vi "AnalysisCompleted.vi"(0 "SystemEvents in":refnum<class "SystemEvents.lvclass">, 1 "event data":variant, 5 "error in (no error)":errorcluster) -> (14 "SystemEvents out":refnum<class "SystemEvents.lvclass">, 19 "error out":errorcluster)   [LabVIEW 2017, in "SystemEvents.lvclass"]
doc: "Fires the Analysis completed event."
uses:
  SystemEvents.lvclass
  SystemEvents.lvclass/SystemEvents.ctl
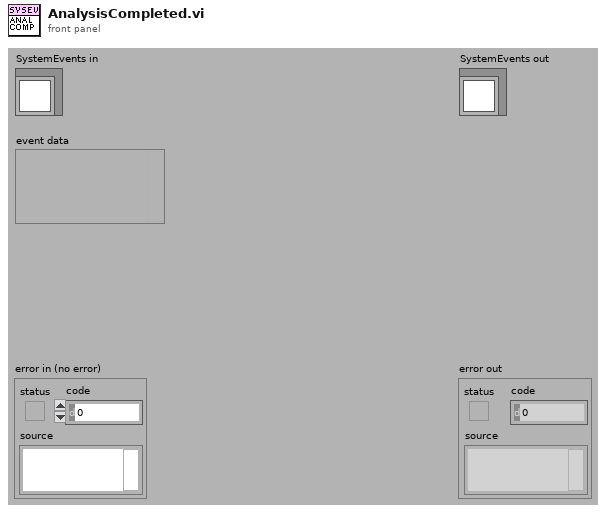
[diagram p1: front panel]
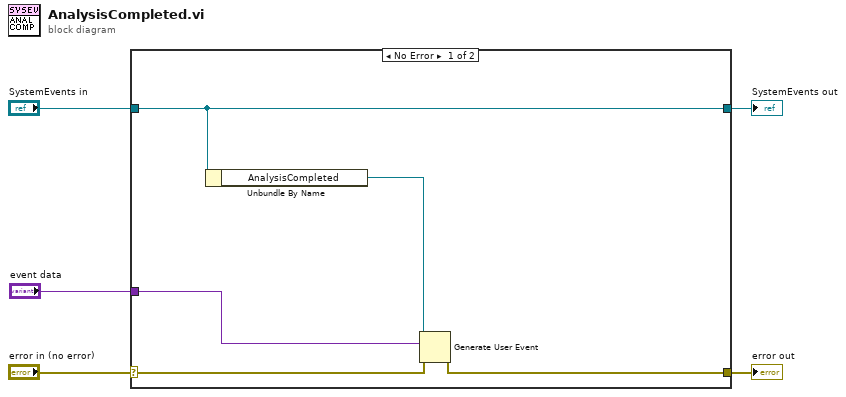
[diagram p0: block diagram]
diagram:
  n1 = case shown="No Error" "error in (no error)" {
    selector: "error in (no error)" -> [w9 w12]
    tunnel: [w8 w12] -> w4
    tunnel: [w10 w11] -> w2
    tunnel: "SystemEvents in" -> [w10 w11]
    tunnel: "event data" -> [w6 _]
    frame No Error {
      n2 = Unbundle By Name(w10) -> ("AnalysisCompleted"=w7:refnum<user-event>)
      n3 = Generate User Event(user event=w7, event data cluster=w6, error in=w9) -> (error out=w8:errorcluster)  [unwired: 1 in, 1 out]
    }
    frame Error {
    }
  }
  "error out" <- w4
  "SystemEvents out" <- w2
